vi "set_hot_cold_colors.vi"(8 "error in (no error)":errorcluster, 9 "color higher limit":u32(colorbox)=16711680, 10 "color lower limit":u32(colorbox)=16711680, 11 "ColorOverlay in":refnum<class "ColorOverlay.lvclass">) -> (0 "error out":errorcluster, 3 "ColorOverlay out":refnum<class "ColorOverlay.lvclass">)   [LabVIEW 2010, in "ColorOverlay.lvclass"]
uses:
  ColorOverlay.lvclass
  ColorOverlay.lvclass/ColorOverlay.ctl
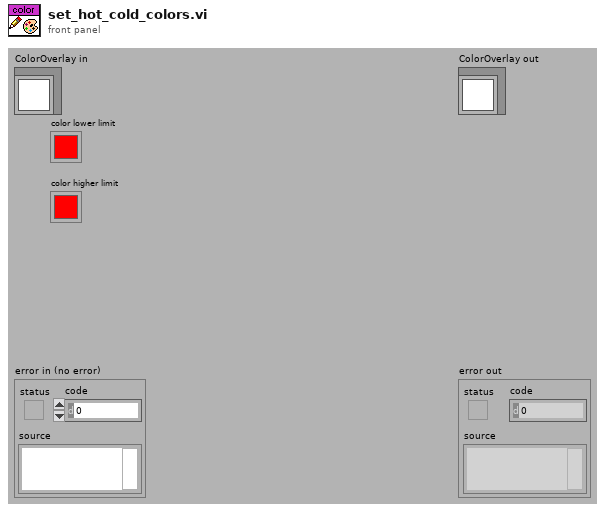
[diagram p1: front panel]
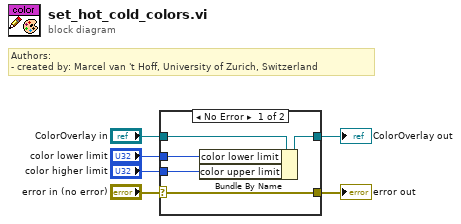
[diagram p0: block diagram]
diagram:
  # "Authors: \n- created by: Marcel van 't Hoff, University of Zurich, Switzerland"
  n1 = case shown="No Error" "error in (no error)" {
    selector: "error in (no error)" -> [w11 w13]
    tunnel: [w11 w13] -> w5
    tunnel: [w9 w12] -> w3
    tunnel: "ColorOverlay in" -> [w10 w12]
    tunnel: "color lower limit" -> [w8 _]
    tunnel: "color higher limit" -> [w7 _]
    frame No Error {
      n2 = Bundle By Name(cluster=w10, "color lower limit"=w8, "color upper limit"=w7) -> (w9:refnum<class "ColorOverlay.lvclass">)
    }
    frame Error {
    }
  }
  "error out" <- w5
  "ColorOverlay out" <- w3
